vi "Wing coordinate sorter.vi"() -> ()   [LabVIEW 2015]
panel:
  out "Sensor no. wing":sgl[](array[numeric])=[2.0, 0.0, 13.0, 12.0, 11.0, 10.0, 6.0, 9.0, 5.0, 8.0, 7.0, 4.0, 21.0, 3.0, 20.0, 19.0, 18.0, 17.0, 16.0, 15.0, 14.0, 1.0]
  out "Sensor no. flap":sgl[](array[numeric])=[22.0, 23.0, 25.0, 26.0, 28.0, 29.0, 27.0, 24.0]
  out "Tube no. wing":sgl[](array[numeric])=[3.0, 1.0, 16.0, 15.0, 14.0, 13.0, 8.0, 12.0, 7.0, 11.0, 9.0, 6.0, 24.0, 5.0, 23.0, 22.0, 21.0, 20.0, 19.0, 18.0, 17.0, 2.0]
  out "Tube no. flap":sgl[](array[numeric])=[25.0, 26.0, 28.0, 29.0, 31.0, 32.0, 30.0, 27.0]
  out "Winding no. wing":sgl[](array[numeric])=[0.0, 1.0, 2.0, 3.0, 4.0, 5.0, 6.0, 7.0, 8.0, 9.0, 10.0, 11.0, 12.0, 13.0, 14.0, 15.0, 16.0, 17.0, 18.0, 19.0, 20.0, 21.0]
  out "Winding no. flap":sgl[](array[numeric])=[0.0, 1.0, 2.0, 3.0, 4.0, 5.0, 6.0, 7.0]
  out "y/c flap":sgl[](array[numeric])=[0.3702977, 0.27414677, 0.19456363, 0.14230296, 0.12718599, 0.15663312, 0.19359294, 0.247963]
  out "y/c wing":sgl[](array[numeric])=[-0.055548523, -0.12028768, -0.124059446, -0.11144002, -0.08997261, -0.06635858, -0.048627622, -0.043094855, -0.034690067, -0.022772176, -0.001057558, 0.02325355, 0.025220403, 0.02517618, 0.023960816, 0.020169007, 0.01457642, -0.00389553, -0.028557567, -0.043236114, -0.04890474, -0.03931195]
  out "x/c flap":sgl[](array[numeric])=[0.9951131, 0.9789507, 0.94671166, 0.898568, 0.83493316, 0.80438995, 0.83493316, 0.9005628]
  out "FLAP: Tube Sorted array":sgl[][](array[numeric])=[[22.0, 25.0, 0.0, 0.9951131, 0.3702977], [23.0, 26.0, 1.0, 0.9789507, 0.27414677], [25.0, 28.0, 2.0, 0.94671166, 0.19456363], [26.0, 29.0, 3.0, 0.898568, 0.14230296], [28.0, 31.0, 4.0, 0.83493316, 0.12718599], [29.0, 32.0, 5.0, 0.80438995, 0.15663312], [27.0, 30.0, 6.0, 0.83493316, 0.19359294], [24.0, 27.0, 7.0, 0.9005628, 0.247963]]
  out "x/c wing":sgl[](array[numeric])=[0.7367813, 0.48221973, 0.35498825, 0.23053746, 0.1323952, 0.06888126, 0.037189517, 0.029719163, 0.020091694, 0.008870252, 1.91e-05, 0.017702324, 0.027253436, 0.03684909, 0.046428833, 0.065556504, 0.08735989, 0.15782876, 0.28504115, 0.412279, 0.5395105, 0.6667451]
  out "WING: Tube sorted array":sgl[][](array[numeric])=[[2.0, 3.0, 0.0, 0.7367813, -0.055548523], [0.0, 1.0, 1.0, 0.48221973, -0.12028768], [13.0, 16.0, 2.0, 0.35498825, -0.124059446], [12.0, 15.0, 3.0, 0.23053746, -0.11144002], [11.0, 14.0, 4.0, 0.1323952, -0.08997261], [10.0, 13.0, 5.0, 0.06888126, -0.06635858], [6.0, 8.0, 6.0, 0.037189517, -0.048627622], [9.0, 12.0, 7.0, 0.029719163, -0.043094855], [5.0, 7.0, 8.0, 0.020091694, -0.034690067], [8.0, 11.0, 9.0, 0.008870252, -0.022772176], [7.0, 9.0, 10.0, 1.91e-05, -0.001057558], [4.0, 6.0, 11.0, 0.017702324, 0.02325355], [21.0, 24.0, 12.0, 0.027253436, 0.025220403], [3.0, 5.0, 13.0, 0.03684909, 0.02517618], [20.0, 23.0, 14.0, 0.046428833, 0.023960816], [19.0, 22.0, 15.0, 0.065556504, 0.020169007], [18.0, 21.0, 16.0, 0.08735989, 0.01457642], [17.0, 20.0, 17.0, 0.15782876, -0.00389553], [16.0, 19.0, 18.0, 0.28504115, -0.028557567], [15.0, 18.0, 19.0, 0.412279, -0.043236114], [14.0, 17.0, 20.0, 0.5395105, -0.04890474], [1.0, 2.0, 21.0, 0.6667451, -0.03931195]]
  in  "FLAP: Sensor no.; Tube no.; Winding no.; x/c; y/c":string="22\t25\t0\t0.995113089\t0.370297701\n23\t26\t1\t0.97895065\t0.274146779\n24\t27\t7\t0.900562822\t0.247962992\n25\t28\t2\t0.946711675\t0.19456363\n26\t29\t3\t0.89856797\t0.142302957\n27\t30\t6\t0.834933139\t0.193592929\n28\t31\t4\t0.834933139\t0.127185986\n29\t32\t5\t0.804389947\t0.156633122\n"
  in  "WING: Sensor no.; Tube no.; Winding no.; x/c; y/c":string="0\t1\t1\t0.482219726\t-0.120287679\n1\t2\t21\t0.666745146\t-0.039311951\n2\t3\t0\t0.73678132\t-0.055548521\n3\t5\t13\t0.036849088\t0.02517618\n4\t6\t11\t0.017702325\t0.02325355\n5\t7\t8\t0.020091693\t-0.034690066\n6\t8\t6\t0.037189517\t-0.048627624\n7\t9\t10\t0.0000191\t-0.001057558\n8\t11\t9\t0.008870252\t-0.022772176\n9\t12\t7\t0.029719162\t-0.043094853\n10\t13\t5\t0.06888126\t-0.066358583\n11\t14\t4\t0.132395191\t-0.089972607\n12\t15\t3\t0.230537465\t-0.111440016\n13\t16\t2\t0.354988244\t-0.124059445\n14\t17\t20\t0.539510482\t-0.04890474\n15\t18\t19\t0.412278999\t-0.043236115\n16\t19\t18\t0.285041154\t-0.028557566\n17\t20\t17\t0.157828761\t-0.00389553\n18\t21\t16\t0.087359891\t0.01457642\n19\t22\t15\t0.065556506\t0.020169006\n20\t23\t14\t0.046428833\t0.023960816\n21\t24\t12\t0.027253435\t0.025220404\n"
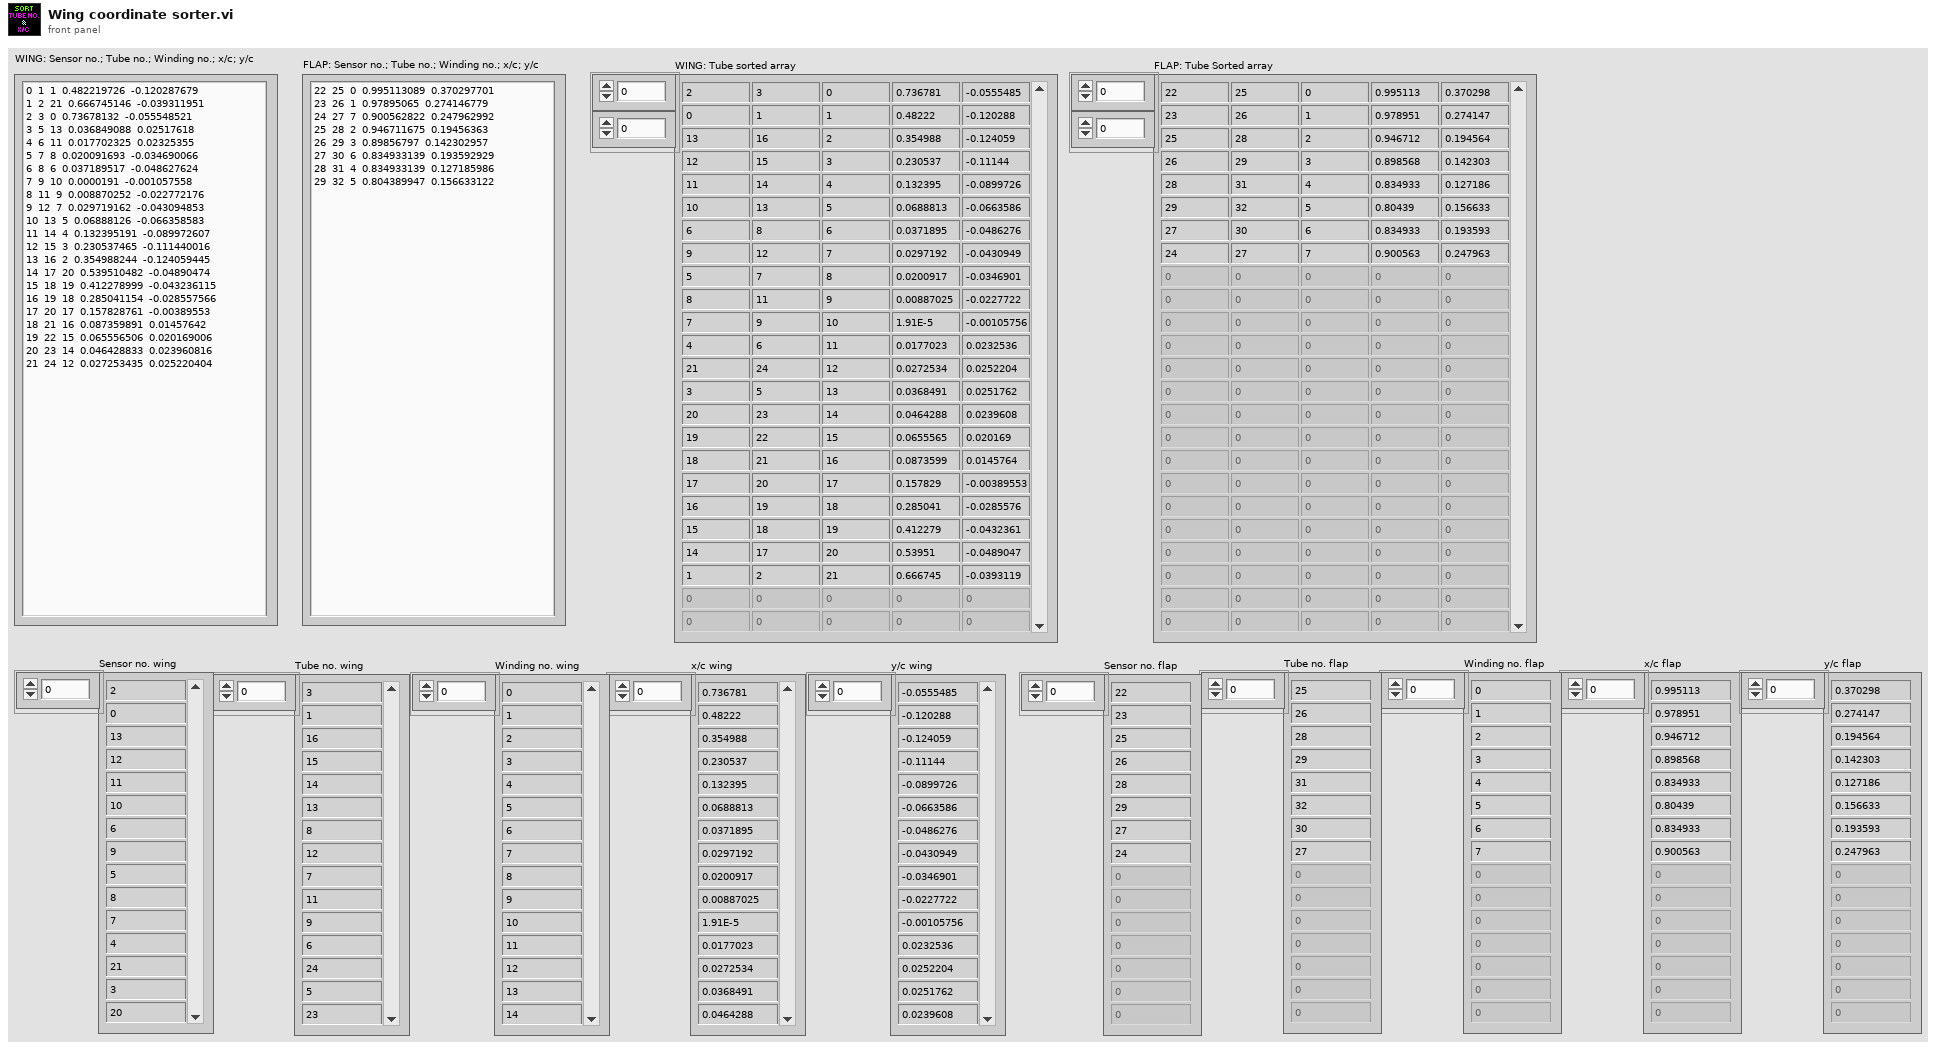
[diagram p1: front panel]
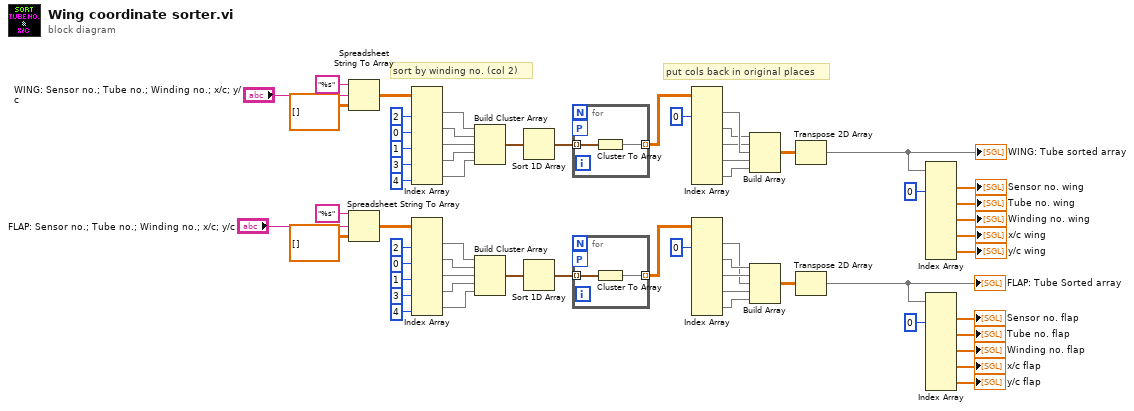
[diagram p0: block diagram]
diagram:
  # "sort by winding no. (col 2)"
  # "put cols back in original places"
  n1 = Spreadsheet String To Array(format string="%s", spreadsheet string="WING: Sensor no.; Tube no.; Winding no.; x/c; y/c", array type (2D Dbl)=sgl[][] []) -> (array=w60:sgl[][])  [unwired: 1 in]
  n2 = Spreadsheet String To Array(format string="%s", spreadsheet string="FLAP: Sensor no.; Tube no.; Winding no.; x/c; y/c", array type (2D Dbl)=sgl[][] []) -> (array=w47:sgl[][])  [unwired: 1 in]
  n3 = Index Array(array=w60, index (col) #1=2 ("disabled index (col)"), index (col) #2=0 ("index (col)"), index (col) #3=1 ("index (col)"), index (col) #4=3 ("index (col)"), index (col) #5=4 ("index (col)")) -> (element #1=w58:sgl[], element #2=w57:sgl[], element #3=w42:sgl[], element #4=w40:sgl[], element #5=w39:sgl[])  [unwired: 5 in]
  n4 = Index Array(array=w47, index (col) #1=2 ("disabled index (col)"), index (col) #2=0 ("index (col)"), index (col) #3=1 ("index (col)"), index (col) #4=3 ("index (col)"), index (col) #5=4 ("index (col)")) -> (element #1=w49:sgl[], element #2=w50:sgl[], element #3=w41:sgl[], element #4=w38:sgl[], element #5=w37:sgl[])  [unwired: 5 in]
  n5 = Build Cluster Array(w58, w57, w42, w40, w39) -> (w56:cluster{sgl, sgl, sgl, sgl, sgl}[])
  n6 = Build Cluster Array(w49, w50, w41, w38, w37) -> (w51:cluster{sgl, sgl, sgl, sgl, sgl}[])
  n7 = Sort 1D Array(array=w56) -> (sorted array=w55:cluster{sgl, sgl, sgl, sgl, sgl}[])
  n8 = Sort 1D Array(array=w51) -> (sorted array=w52:cluster{sgl, sgl, sgl, sgl, sgl}[])
  n9 = for {
    tunnel: w55 -> [w64] mode=indexing
    tunnel: [w63] -> w27 mode=indexing
    workers-P: _ -> [_]
    n10 = Cluster To Array(cluster=w64) -> (array=w63:sgl[])
  }
  n11 = for {
    tunnel: w52 -> [w66] mode=indexing
    tunnel: [w65] -> w14 mode=indexing
    workers-P: _ -> [_]
    n12 = Cluster To Array(cluster=w66) -> (array=w65:sgl[])
  }
  n13 = Index Array(array=w27, index (col) #1=0 ("disabled index (col)")) -> (element #1=w26:sgl[], element #2=w25:sgl[], element #3=w24:sgl[], element #4=w23:sgl[], element #5=w22:sgl[])  [unwired: 9 in]
  n14 = Index Array(array=w14, index (col) #1=0 ("disabled index (col)")) -> (element #1=w16:sgl[], element #2=w17:sgl[], element #3=w18:sgl[], element #4=w19:sgl[], element #5=w20:sgl[])  [unwired: 9 in]
  n15 = Build Array(w25, w24, w26, w23, w22) -> (w21:sgl[][])
  n16 = Build Array(w17, w18, w16, w19, w20) -> (w13:sgl[][])
  n17 = Transpose 2D Array(2D array=w21) -> (transposed array=w12:sgl[][])
  "WING: Tube sorted array" <- w12
  n18 = Transpose 2D Array(2D array=w13) -> (transposed array=w11:sgl[][])
  "FLAP: Tube Sorted array" <- w11
  n19 = Index Array(array=w12, index (col) #1=0 ("disabled index (col)")) -> (element #1=→"Sensor no. wing":sgl[], element #2=→"Tube no. wing":sgl[], element #3=→"Winding no. wing":sgl[], element #4=→"x/c wing":sgl[], element #5=→"y/c wing":sgl[])  [unwired: 9 in]
  n20 = Index Array(array=w11, index (col) #1=0 ("disabled index (col)")) -> (element #1=→"Sensor no. flap":sgl[], element #2=→"Tube no. flap":sgl[], element #3=→"Winding no. flap":sgl[], element #4=→"x/c flap":sgl[], element #5=→"y/c flap":sgl[])  [unwired: 9 in]
